vi "Global 2.vi"() -> ()   [LabVIEW 2024]
panel:
  in  "Test Done":bool
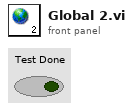
[diagram p1: front panel]
diagram:
